vi "IV_Reverse.vi"(3 "error in (no error)":errorcluster, 4 "Input cluster":T1={"Vmin"=0.001, "Vmax"=0.001, "Step"=0.001, "milliseconds to wait"=10, "limit current [mA]"=0.001, "ms to ramp down"=10, "Stop"=FALSE} {"Step" format="%#_13g"; "Vmax" format="%#_13g"}, 5 "Upper Measurement Range":u16(ring)=2 items=["20mA", "2mA", "200uA", "20uA", "2uA", "200nA", "20nA", "2nA"], 6 "VISA resource name in":refnum<visa-resource-name>) -> (0 "error out":errorcluster, 1 "IV cluster":cluster{dbl[], dbl[]}, 2 "VISA resource name out":refnum<visa-resource-name>)   [LabVIEW 2022 SP3]
uses:
  IV_cluster_in.ctl
  <instrlib>/Keithley 648X Series/Keithley 648X Series.lvlib
panel:
  out "XY Graph 2":cluster{dbl[], dbl[]}(graph)
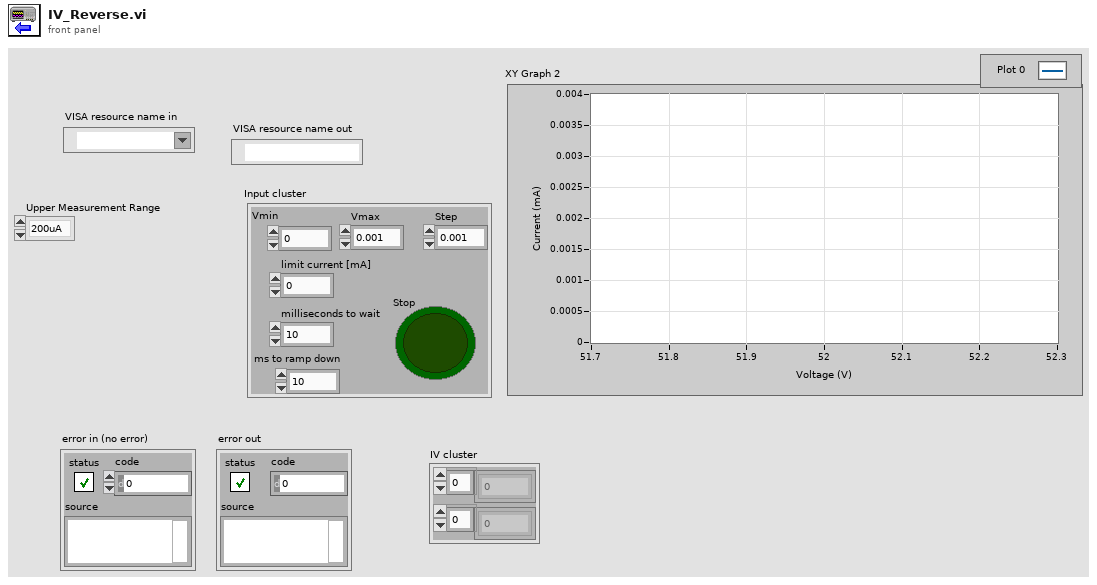
[diagram p1: front panel]
types:
  T1 = typedef "IV_cluster_in.ctl" = cluster{"Vmin":dbl, "Vmax":dbl, "Step":dbl, "milliseconds to wait":u32, "limit current [mA]":dbl, "ms to ramp down":u32, "Stop":bool}
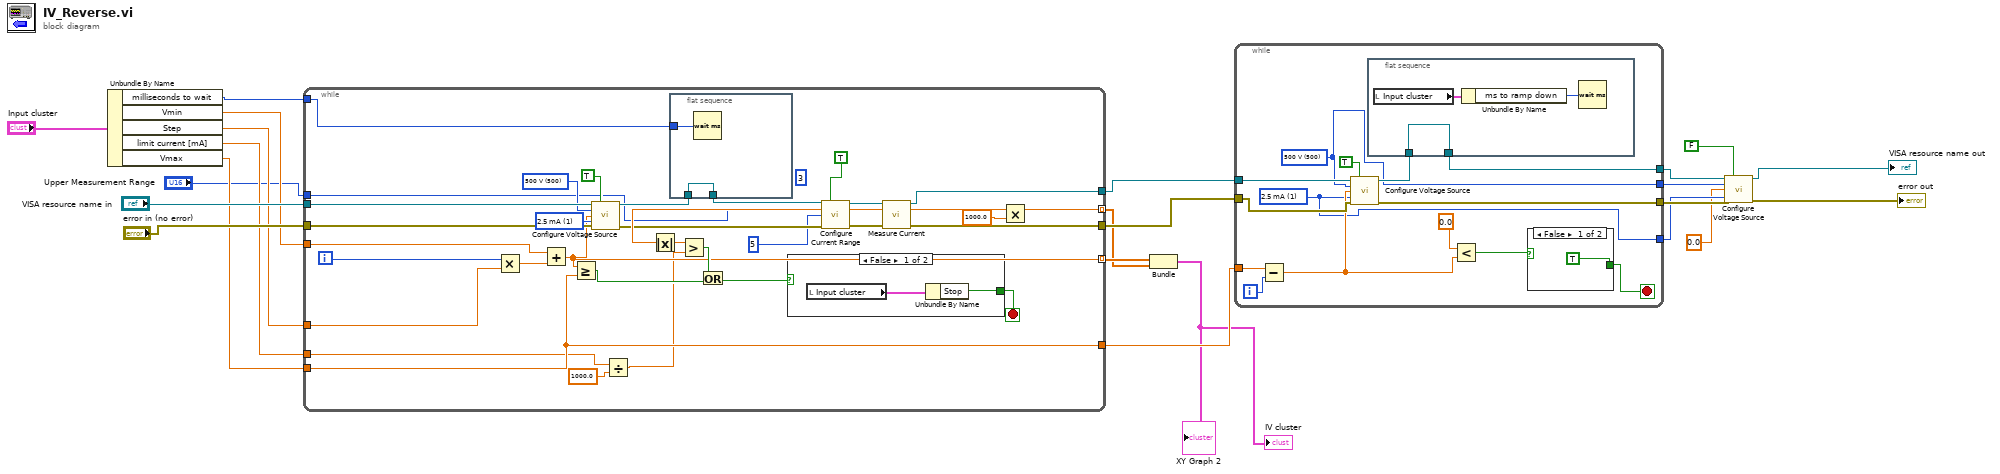
[diagram p0: block diagram]
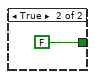
[diagram p2: hidden frame]
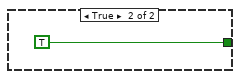
[diagram p3: hidden frame]
diagram:
  n1 = Unbundle By Name("Input cluster") -> ("milliseconds to wait"=w15:u32, "Vmin"=w14:dbl, "Step"=w13:dbl, "limit current [mA]"=w12:dbl, "Vmax"=w11:dbl)
  n2 = while {
    tunnel: [w40] -> w19 mode=indexing
    tunnel: [w56] -> w21
    tunnel: [w55] -> w22
    tunnel: "VISA resource name in" -> [w54]
    tunnel: "error in (no error)" -> [w53]
    tunnel: w14 -> [w52]
    tunnel: [w41] -> w20 mode=indexing
    tunnel: [w36] -> w23
    tunnel: w15 -> [w38]
    tunnel: w13 -> [w37]
    tunnel: w12 -> [w35]
    tunnel: w11 -> [w36]
    tunnel: "Upper Measurement Range" -> [w24]
    i -> [w43]
    stop <- w48 stop-if-true
    (unwired) i16 3
    w50 = u16 500 items=["10 V"=10, "50 V"=50, "500 V"=500] ("Voltage Source Range (10 V)")
    w51 = u16 1 items=["25 mA", "2.5 mA", "250 uA", "25 uA"] ("Current Limit (25 mA)")
    n3 = Multiply(x=w43, y=w37) -> (x*y=w44:dbl)
    n4 = Add(x=w52, y=w44) -> (x+y=w41:dbl)
    n5 = Greater Or Equal?(x=w41, y=w36) -> (x >= y?=w46:bool)
    n6 = call <instrlib>:"Configure Voltage Source.vi"("VISA resource name"=w54, "Enable Voltage Source (F: Disable)"=TRUE, "Voltage Source Range (10 V)"=w50, "Voltage Level (0 V)"=w41, "Current Limit (25 mA)"=w51, "error in (no error)"=w53) -> ("VISA resource name out"=w42:refnum<visa-resource-name>, "error out"=w27:errorcluster)  [unwired: 8 in]
    n7 = Divide(x=w35, y=1000.0) -> (x/y=w34:dbl)
    n8 = flat-sequence {
      tunnel: w42 -> [w58]
      tunnel: [w58] -> w28
      tunnel: w38 -> [w57]
      frame #0 {
        n9 = Wait (ms)(milliseconds to wait=w57) -> ()  [unwired: 1 out]
      }
    }
    n10 = call <instrlib>:"Configure Current Range.vi"("VISA resource name"=w28, "Autorange (T: Enable)"=TRUE, "Auto Range Max (20mA)"=w24, "Auto Range Min (2nA)"=i16 5, "error in (no error)"=w27) -> ("VISA resource name out"=w30:refnum<visa-resource-name>, "error out"=w29:errorcluster)  [unwired: 9 in]
    n11 = call <instrlib>:"Measure Current.vi"("VISA resource name"=w30, "error in (no error)"=w29) -> ("VISA resource name out"=w56:refnum<visa-resource-name>, "Measurement"=w32:dbl, "error out"=w55:errorcluster)  [unwired: 11 in]
    n12 = Absolute Value(x=w32) -> (abs(x)=w31:dbl)
    n13 = Greater?(x=w31, y=w34) -> (0:w49:bool)
    n14 = Or(x=w49, y=w46) -> (x .or. y?=w47:bool)
    n15 = case shown="False" w47 {
      tunnel: [w59 TRUE] -> w48
      frame False {
        n16 = local read "Input cluster"() -> (w60:T1)
        n17 = Unbundle By Name(w60) -> ("Stop"=w59:bool)
      }
      frame True {
      }
    }
    n18 = Multiply(x=w32, y=1000.0) -> (x*y=w40:dbl)
  }
  n19 = Bundle(w20, w19) -> (→"XY Graph 2" →"IV cluster":cluster{dbl[], dbl[]})  [unwired: 1 in]
  n20 = while {
    tunnel: w21 -> [w73]
    tunnel: [w64] -> w9
    tunnel: w22 -> [w72]
    tunnel: [w71] -> w8
    tunnel: w23 -> [w66]
    tunnel: [w63] -> w5
    tunnel: [w62] -> w4
    i -> [w75]
    stop <- w67 stop-if-true
    w63 = u16 500 items=["10 V"=10, "50 V"=50, "500 V"=500] ("Voltage Source Range (10 V)")
    w62 = u16 1 items=["25 mA", "2.5 mA", "250 uA", "25 uA"] ("Current Limit (25 mA)")
    n21 = Subtract(x=w66, y=w75) -> (x-y=w69:dbl)
    n22 = call <instrlib>:"Configure Voltage Source.vi"("VISA resource name"=w73, "Enable Voltage Source (F: Disable)"=TRUE, "Voltage Source Range (10 V)"=w63, "Voltage Level (0 V)"=w69, "Current Limit (25 mA)"=w62, "error in (no error)"=w72) -> ("VISA resource name out"=w65:refnum<visa-resource-name>, "error out"=w71:errorcluster)  [unwired: 8 in]
    n23 = flat-sequence {
      tunnel: w65 -> [w77]
      tunnel: [w77] -> w64
      frame #0 {
        n24 = local read "Input cluster"() -> (w78:T1)
        n25 = Unbundle By Name(w78) -> ("ms to ramp down"=w76:u32)
        n26 = Wait (ms)(milliseconds to wait=w76) -> ()  [unwired: 1 out]
      }
    }
    n27 = Less?(x=0.0 ("Step"), y=w69) -> (x < y?=w68:bool)
    n28 = case shown="False" w68 {
      tunnel: [TRUE FALSE] -> w67
      frame False {
      }
      frame True {
      }
    }
  }
  n29 = call <instrlib>:"Configure Voltage Source.vi"("VISA resource name"=w9, "Enable Voltage Source (F: Disable)"=FALSE, "Voltage Source Range (10 V)"=w5, "Voltage Level (0 V)"=0.0, "Current Limit (25 mA)"=w4, "error in (no error)"=w8) -> ("VISA resource name out"=→"VISA resource name out":refnum<visa-resource-name>, "error out"=→"error out":errorcluster)  [unwired: 8 in]
